vi "Test Bench v15 - TDMS.vi"() -> ()   [LabVIEW 2022 SP3]
uses:
  WhiteNoise.ctl
  <vilib>/Utility/error.llb/DialogType.ctl
  <vilib>/Platform/TimedLoop/XDataNode/timing_clust.ctl
  <vilib>/Platform/TimedLoop/XDataNode/nitl_modes.ctl
  <vilib>/Platform/TimedLoop/XDataNode/wakeup.ctl
  <vilib>/DAQmx/write.llb/DAQmx Write (Analog 2D DBL NChan NSamp).vi
  <vilib>/DAQmx/read.llb/DAQmx Read (Analog 1D DBL 1Chan NSamp).vi
  <vilib>/DAQmx/create/channels.llb/DAQmx Create Channel (AI-Acceleration-Accelerometer).vi
  <vilib>/DAQmx/configure/timing.llb/DAQmx Timing (Sample Clock).vi
  <vilib>/DAQmx/miscellaneous.llb/DAQmx Fill In Error Info.vi
  <vilib>/platform/TimedLoop/XDataNode/XDataNode.xnode
  <vilib>/DAQmx/create/channels.llb/DAQmx Create Channel (AO-Voltage-Basic).vi
  <resource>/objmgr/daqmx.rc
  <vilib>/measure/NI_MABase.lvlib
  <vilib>/Platform/TimedLoop/XDataNode/XDNodeRunTimeDep.lvlib
  <vilib>/Platform/TimedLoop/TimeConversion.llb/rt-milliseconds-to-timestamp.vi
panel:
  in  "stop":bool
  out "x/y":dbl
  out "SampClk.Rate":dbl
  out "Accel. 1 Raw":dbl[](graph)
  in  "Enable Display":bool=TRUE
  in  "Folder to save file to":path=path "C:/Users/LAV-UFSC-2023/Documents/LAV-TCC/Dados-Experimentos/Dados-Bancada-LABVIEW"
  out "Output Signal":dynamicdata(graph)
  in  "Accel. 2":bool
  out "New file path":path
  in  "Signal Output\nControl":enum32{"White Noise", "Harmonic"}(tab)
  in  "White Noise\nParameters":T2={"Seed"=0.0, "Standard Deviation"=0.2, "Reset"=FALSE, "Iterator"=1.0, "Seed"=-1, "Lower Cut-Off"=5.0, "Upper Cut-Off"=350.0} {"Upper Cut-Off" min=5.0 max=350.0 step=10.0; "Lower Cut-Off" min=5.0 max=350.0 step=10.0; "Standard Deviation" min=0.001 max=3.0 step=0.05 format="%0.2p"}
  out "dt White Noise":dbl
  in  "Hamonic\nParameters":T3={"Waveform Type"=0, "Frequency"=10.0, "Amplitude"=0.25} {"Frequency" min=5.0 max=350.0 step=10.0 format="%0.2p"; "Waveform Type" items=["Sine Wave", "Triangle Wave", "Square Wave", "Sawtooth Wave"]; "Amplitude" min=0.001 max=0.3 step=0.05 format="%0.2p"}
  out "dt Harmonic":dbl
  in  "Output":bool=TRUE
  # "Filter"
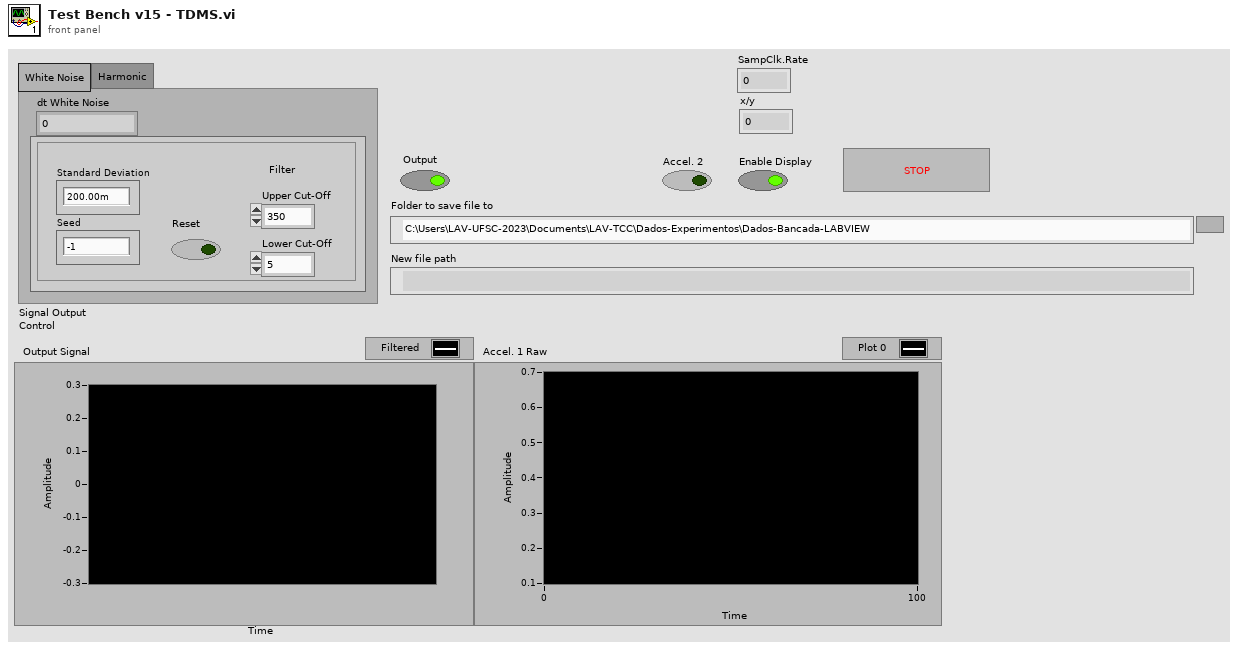
[diagram p1: front panel]
types:
  T1 = typedef "WhiteNoise.ctl" = dbl
  T2 = cluster{"Seed":T1, "Standard Deviation":dbl, "Reset":bool, "Iterator":dbl, "Seed":i8, "Lower Cut-Off":dbl, "Upper Cut-Off":dbl}
  T3 = cluster{"Waveform Type":u16, "Frequency":dbl, "Amplitude":dbl}
  T4 = typedef "DialogType.ctl" = u16
  T5 = enum16{"open", "open or create", "create or replace", "create", "open (read-only)"}
  T6 = typedef "XDNodeRunTimeDep.lvlib/timing_clust.ctl" = cluster{"Expected End [f-1]":u64, "Actual End [f-1]":u64, "Finished Late? [f-1]":bool, "Expected End [i-1]":u64, "Actual End [i-1]":u64, "Finished Late? [i-1]":bool, "Expected Start [i]":u64, "Actual Start [i]":u64, "Expected Start [f]":u64, "Actual Start [f]":u64, "Source Name":string, "Structure Name":string, "Period":i64, "Deadline":i64, "Offset":i64, "Start":i64, "Priority":i32, "Timeout":i32, "Mode":T7, "Wakeup Reason":T8, "Error":errorcluster, "Source Type":string, "Secondary Source Type":string, "Global End Time":u64, "Global Start Time":u64, "Frame Duration":u64, "Iteration Duration":u64, "Assigned CPU":i32, "I/O Scan Engine Mode":u32}
  T7 = typedef "XDNodeRunTimeDep.lvlib/nitl_modes.ctl" = enum32{"No Change", "Process missed periods, maintain original phase", "Discard missed periods, maintain original phase", "Process missed periods, ignore original phase", "Discard missed periods, ignore original phase"}
  T8 = typedef "XDNodeRunTimeDep.lvlib/wakeup.ctl" = enum32{"Normal", "Aborted", "Asynchronous wakeup", "Timing source error", "Timed loop error", "Timeout"}
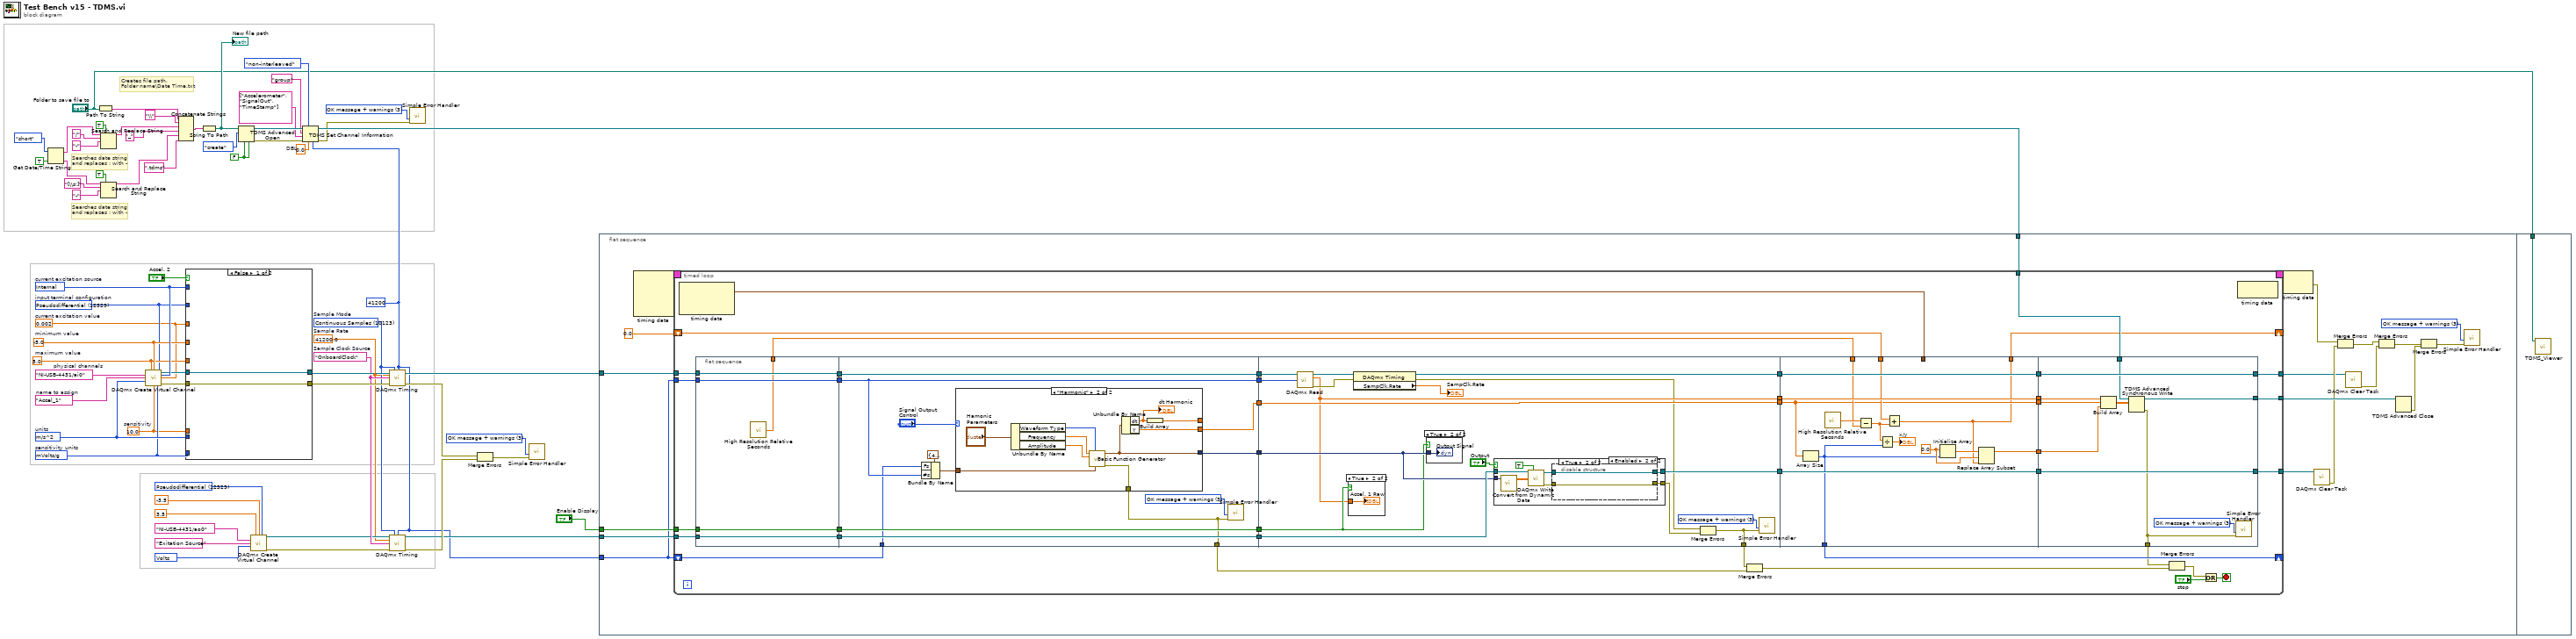
[diagram p0: block diagram]
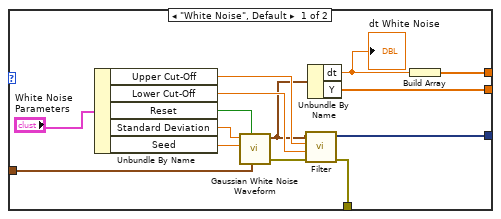
[diagram p2: hidden frame]
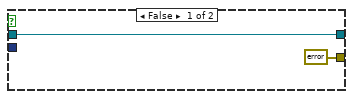
[diagram p5: hidden frame]
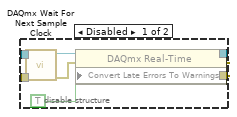
[diagram p6: hidden frame]
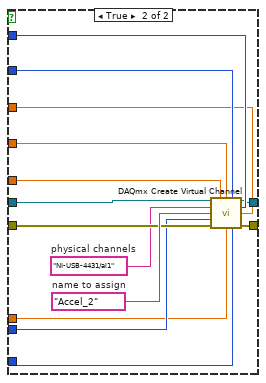
[diagram p7: hidden frame]
diagram:
  w4 = T4 3 items=["no dialog", "OK message", "continue or stop message", "OK message + warnings", "continue/stop + warnings"] ("type of dialog (OK msg:1)")
  w1 = 41200 ("samples per channel")
  w9 = 0.0  # DBL
  w11 = FALSE ("enable asynchronous? (T)")
  w7 = T4 3 items=["no dialog", "OK message", "continue or stop message", "OK message + warnings", "continue/stop + warnings"] ("type of dialog (OK msg:1)")
  w51 = 12529 items=["Default"=-1, "RSE"=10083, "Differential"=10106, "Pseudodifferential"=12529] ("output terminal configuration")
  w49 = 10348 items=["Volts"=10348, "From Custom Scale"=10065] ("units")
  w55 = 12509 items=["mVolts/g"=12509, "Volts/g"=12510]  # sensitivity units
  w46 = 10.0  # sensitivity
  w54 = 0.002  # current excitation value
  w62 = 10200 items=["Internal"=10200, "External"=10167, "None"=10230]  # current excitation source
  w56 = tag "NI-USB-4431/ai0"  # physical channels
  w43 = tag "OnboardClock"  # Sample Clock Source
  w6 = 41200.0  # Sample Rate
  w42 = 10123 items=["Finite Samples"=10178, "Continuous Samples"=10123, "Hardware Timed Single Point"=12522]  # Sample Mode
  w58 = 12529 items=["default"=-1, "RSE"=10083, "NRSE"=10078, "Differential"=10106, "Pseudodifferential"=12529]  # input terminal configuration
  w61 = -5.0  # minimum value
  w60 = 5.0  # maximum value
  w64 = "Accel_1"  # name to assign
  w59 = 12470 items=["g"=10186, "m/s^2"=12470, "in/s^2"=12471, "From Custom Scale"=10065]  # units
  # "Searches date string\nand replaces : with -"
  # "Searches date string\nand replaces : with -"
  # "Creates file path.\nFolder name\\Date Time.txt"
  n1 = Get Date/Time String(date format (0)=enum16{"short", "long", "abbreviated"}."short", want seconds? (F)=TRUE) -> (date string=w19:string, time string=w32:string)  [unwired: 1 in]
  n2 = Path To String(path="Folder to save file to") -> (string=w27:string)
  n3 = Search and Replace String(replace all?=TRUE ("replace all? (F)"), input string=w19, search string="/" ("replace string (\"\")"), replace string="-" ("replace string (\"\")")) -> (result string=w18:string)  [unwired: 4 in, 3 out]
  n4 = Search and Replace String(replace all?=TRUE ("replace all? (F)"), input string=w32, search string="[\\s:]" ("replace string (\"\")"), replace string="-" ("replace string (\"\")")) -> (result string=w25:string)  [unwired: 4 in, 3 out]
  n5 = call-poly <vilib>:"DAQmx Create Virtual Channel.vi"("maximum value"=w60, "minimum value"=w61, "input terminal configuration"=w58, "physical channels"=w56, "current excitation source"=w62, "name to assign"=w64, "current excitation value"=w54, "units"=w59, "sensitivity"=w46, "sensitivity units"=w55) -> ("task out"=w57:refnum<k21>, "error out"=w63:errorcluster)  [unwired: 4 in]
  n6 = Concatenate Strings(w27, "\\" ("string"), w18, "_" ("string"), w25, ".tdms" ("string")) -> (w23:string)
  n7 = case shown="False" "Accel. 2" {
    tunnel: w63 -> [w66 w79]
    tunnel: w62 -> [_ w78]
    tunnel: w61 -> [_ w77]
    tunnel: w60 -> [_ w76]
    tunnel: w59 -> [_ w75]
    tunnel: w58 -> [_ w74]
    tunnel: w57 -> [w65 w73]
    tunnel: w55 -> [_ w71]
    tunnel: w54 -> [_ w70]
    tunnel: w46 -> [_ w69]
    tunnel: [w66 w68] -> w45
    tunnel: [w65 w67] -> w44
    frame False {
    }
    frame True {
      w72 = tag "NI-USB-4431/ai1"  # physical channels
      w80 = "Accel_2"  # name to assign
      n8 = call-poly <vilib>:"DAQmx Create Virtual Channel.vi"("task in"=w73, "maximum value"=w76, "minimum value"=w77, "input terminal configuration"=w74, "physical channels"=w72, "current excitation source"=w78, "name to assign"=w80, "current excitation value"=w70, "units"=w75, "error in"=w79, "sensitivity"=w69, "sensitivity units"=w71) -> ("task out"=w67:refnum<k21>, "error out"=w68:errorcluster)  [unwired: 2 in]
    }
  }
  n9 = String To Path(string=w23) -> (path=w36:path)
  "New file path" <- w36
  n10 = TDMS Advanced Open(4:w11, 6:w11, 10:T5."create" ("operation (0:open)"), 11:w36) -> (0:w15:errorcluster, 3:w14:refnum<k34>)  [unwired: 1 in, 1 out]
  n11 = call-poly <vilib>:"DAQmx Create Virtual Channel.vi"("maximum value"=3.5, "minimum value"=-3.5, "output terminal configuration"=w51, "physical channels"=tag "NI-USB-4431/ao0", "name to assign"="Exitation Source", "units"=w49) -> ("task out"=w40:refnum<k21>, "error out"=w41:errorcluster)  [unwired: 8 in]
  n12 = TDMS Set Channel Information(4:w1, 6:w9, 7:enum16{"non-interleaved", "interleaved"}."non-interleaved" ("data layout (0:non-interleaved)"), 8:w15, 9:string[] ["Accelerometer", "SignalOut", "TimeStamp"] ("channel name(s)"), 10:"group" ("group name (Untitled)"), 11:w14) -> (0:w8:errorcluster, 3:w35:refnum<k34>)
  n13 = call-poly <vilib>:"DAQmx Timing.vi"("task/channels in"=w44, "sample mode"=w42, "samples per channel"=w1, "rate"=w6, "source"=w43, "error in"=w45) -> ("task out"=w3:refnum<k21>, "error out"=w48:errorcluster)  [unwired: 8 in]
  n14 = call-poly <vilib>:"DAQmx Timing.vi"("task/channels in"=w40, "sample mode"=w42, "samples per channel"=w1, "rate"=w6, "source"=w43, "error in"=w41) -> ("task out"=w38:refnum<k21>, "error out"=w39:errorcluster)  [unwired: 8 in]
  n15 = call <vilib>:"Simple Error Handler.vi"("type of dialog (OK msg:1)"=w7, "error in (no error)"=w8) -> ()  [unwired: 3 in, 5 out]
  n16 = Merge Errors(w48, w39) -> (w2:errorcluster)
  n17 = call <vilib>:"Simple Error Handler.vi"("type of dialog (OK msg:1)"=w4, "error in (no error)"=w2) -> ()  [unwired: 3 in, 5 out]
  n18 = flat-sequence {
    tunnel: w38 -> [w96]
    tunnel: w3 -> [w94]
    tunnel: w35 -> [w93]
    tunnel: "Enable Display" -> [w91]
    tunnel: w1 -> [w81]
    tunnel: "Folder to save file to" -> [w250]
    frame #0 {
      w97 = T4 3 items=["no dialog", "OK message", "continue or stop message", "OK message + warnings", "continue/stop + warnings"] ("type of dialog (OK msg:1)")
      n19 = node-c288() -> (w99:T6)  [unwired: 4 in]
      n20 = timed-loop {
        tunnel: w96 -> [w139]
        tunnel: [w137] -> w95
        tunnel: w94 -> [w138]
        tunnel: [w136] -> w88
        tunnel: w93 -> [w112]
        tunnel: [w133] -> w92
        tunnel: w91 -> [w135]
        shift-right: [w108] -> _
        shift-left: w81 -> [w117]
        tunnel: w81 -> [w120]
        timing: w99 -> [_]
        timing-out: [_] -> w98
        shift-right: [w107] -> _
        shift-left: 0.0 -> [w110]
        stop <- w118 stop-if-true
        n21 = node-c288() -> (w111:timestamp)  [unwired: 1 in, 2 out]
        n22 = flat-sequence {
          tunnel: w135 -> [w146]
          tunnel: w138 -> [w147]
          tunnel: w139 -> [w148]
          tunnel: [w148] -> w134
          tunnel: [w147] -> w132
          tunnel: [w146] -> w123
          tunnel: w120 -> [w145]
          tunnel: [w145] -> w119
          tunnel: [w144] -> w109
          tunnel: w134 -> [w156]
          tunnel: [w157] -> w131
          tunnel: [w153] -> w129
          tunnel: w132 -> [w157]
          tunnel: [w156] -> w127
          tunnel: [w154] -> w125
          tunnel: [w155] -> w124
          tunnel: w123 -> [w154]
          tunnel: [w152] -> w121
          tunnel: w119 -> [w152]
          tunnel: w117 -> [w151]
          tunnel: [w150] -> w103
          tunnel: w131 -> [w193]
          tunnel: [w189] -> w130
          tunnel: w129 -> [w201]
          tunnel: [w201] -> w128
          tunnel: w127 -> [w199]
          tunnel: [w198] -> w126
          tunnel: w125 -> [w194]
          tunnel: w124 -> [w197]
          tunnel: [w192] -> w122
          tunnel: w121 -> [w191]
          tunnel: [w185] -> w104
          tunnel: w130 -> [w234]
          tunnel: w128 -> [w230]
          tunnel: w126 -> [w236]
          tunnel: w122 -> [w235]
          tunnel: [w236] -> w116
          tunnel: [w235] -> w115
          tunnel: [w234] -> w114
          tunnel: [w230] -> w113
          tunnel: w111 -> [_]
          tunnel: w110 -> [w231]
          tunnel: w109 -> [w232]
          tunnel: [w223] -> w108
          tunnel: [w225] -> w107
          tunnel: [w226] -> w106
          tunnel: [w242] -> w133
          tunnel: [w245] -> w136
          tunnel: [w246] -> w137
          tunnel: w116 -> [w246]
          tunnel: w115 -> [w245]
          tunnel: w114 -> [w240]
          tunnel: w113 -> [w241]
          tunnel: w112 -> [w243]
          tunnel: w106 -> [w239]
          tunnel: [w237] -> w100
          frame #0 {
            n23 = call <vilib>:"High Resolution Relative Seconds.vi"() -> ("relative seconds"=w144:dbl)
          }
          frame #1 {
            w149 = T4 3 items=["no dialog", "OK message", "continue or stop message", "OK message + warnings", "continue/stop + warnings"] ("type of dialog (OK msg:1)")
            n24 = Bundle By Name(cluster=cluster{"Fs":dbl, "#s":dbl} {"Fs"=41200.0, "#s"=41200.0} ("sampling info"), "Fs"=w151, "#s"=w152) -> (w159:cluster{"Fs":dbl, "#s":dbl})
            n25 = case shown="\"Harmonic\"" "Signal Output\nControl" {
              tunnel: w159 -> [w172 w183]
              tunnel: [w164 w178] -> _
              tunnel: [w163 w177] -> w155
              tunnel: [w162 w176] -> w153
              tunnel: [w161 w175] -> w150
              frame "White Noise", Default {
                n26 = Unbundle By Name("White Noise\nParameters") -> ("Upper Cut-Off"=w168:dbl, "Lower Cut-Off"=w167:dbl, "Reset"=w169:bool, "Standard Deviation"=w170:dbl, "Seed"=w171:T1)
                n27 = call <vilib>:"Gaussian White Noise Waveform.vi"("sampling info"=w172, "reset signal"=w169, "seed"=w171, "standard deviation"=w170) -> ("error out"=w174:errorcluster, "signal out"=w166:waveform(dbl))  [unwired: 6 in]
                n28 = call "Filter"("error in (no error)"=w174, "Lower Cut-Off"=w167, "Upper Cut-Off"=w168, "Signal"=w166) -> ("error out"=w161:errorcluster, "Filtered Signal"=w163:dynamicdata)  [unwired: 6 in]
                n29 = Unbundle By Name(w166) -> ("dt"=w165:dbl, "Y"=w162:dbl[])
                "dt White Noise" <- w165
                n30 = Build Array(w165) -> (w164:dbl[])
              }
              frame "Harmonic" {
                n31 = Unbundle By Name("Hamonic\nParameters") -> ("Waveform Type"=w182:u16, "Frequency"=w181:dbl, "Amplitude"=w180:dbl)
                n32 = call <vilib>:"Basic Function Generator.vi"("sampling info"=w183, "signal type"=w182, "amplitude"=w180, "frequency"=w181) -> ("error out"=w175:errorcluster, "signal out"=w177:waveform(dbl))  [unwired: 5 in, 1 out]
                n33 = Unbundle By Name(w177) -> ("dt"=w179:dbl, "Y"=w176:dbl[])
                "dt Harmonic" <- w179
                n34 = Build Array(w179) -> (w178:dbl[])
              }
            }
            n35 = call <vilib>:"Simple Error Handler.vi"("type of dialog (OK msg:1)"=w149, "error in (no error)"=w150) -> ()  [unwired: 3 in, 5 out]
          }
          frame #2 {
            w188 = T4 3 items=["no dialog", "OK message", "continue or stop message", "OK message + warnings", "continue/stop + warnings"] ("type of dialog (OK msg:1)")
            n36 = call-poly <vilib>:"DAQmx Read.vi"("task/channels in"=w193, "number of samples per channel"=w191) -> ("task out"=w195:refnum<k21>, "data"=w189:dbl[], "error out"=w196:errorcluster)  [unwired: 11 in]
            n37 = case shown="True" w194 {
              tunnel: w189 -> [_ w202]
              frame False {
              }
              frame True {
                "Accel. 1 Raw" <- w202
              }
            }
            n38 = property class="DAQmx Timing"(reference=w195, error in=w196) -> (reference out=w192:refnum<k21>, error out=w187:errorcluster, "SampClk.Rate"=→"SampClk.Rate":dbl)
            n39 = case shown="True" w194 {
              tunnel: w197 -> [_ w203]
              frame False {
              }
              frame True {
                "Output Signal" <- w203
              }
            }
            n40 = case shown="True" "Output" {
              tunnel: w199 -> [w205 w213]
              tunnel: [errorcluster {"status"=FALSE, "code"=0, "source"=""} ("error out") w209] -> w186
              tunnel: [w205 w210] -> w198
              tunnel: w197 -> [_ w208]
              frame False {
              }
              frame True {
                n41 = call "Convert from Dynamic Data"("Dynamic Data Type"=w208) -> ("Array"=w207:dbl[][])  [unwired: 3 in]
                n42 = call-poly <vilib>:"DAQmx Write.vi"("task/channels in"=w213, "auto start"=TRUE, "data"=w207) -> ("task out"=w212:refnum<k21>, "error out"=w211:errorcluster)  [unwired: 10 in, 1 out]
                n43 = disable-structure shown="Enabled" {
                  disable-tunnel: w212 -> [w220 w221]
                  disable-tunnel: w211 -> [w219 w222]
                  disable-tunnel: [w217 w221] -> w210
                  disable-tunnel: [w216 w222] -> w209
                  frame Disabled {
                    n44 = call <vilib>:"DAQmx Wait For Next Sample Clock.vi"("task/channels in"=w220, "error in"=w219) -> ("task out"=w218:refnum<k21>, "error out"=w215:errorcluster)  [unwired: 11 in, 1 out]
                    n45 = property class="DAQmx Real-Time"(reference=w218, error in=w215, "Convert Late Errors To Warnings"=TRUE ("ConvLateErrorsToWarnings")) -> (reference out=w217:refnum<k21>, error out=w216:errorcluster)
                  }
                  frame Enabled {
                  }
                }
              }
            }
            n46 = Merge Errors(w187, w186) -> (w185:errorcluster)
            n47 = call <vilib>:"Simple Error Handler.vi"("type of dialog (OK msg:1)"=w188, "error in (no error)"=w185) -> ()  [unwired: 3 in, 5 out]
          }
          frame #3 {
            w227 = 0.0 ("element")
            n48 = Array Size(array=w230) -> (size(s)=w223:i32)
            n49 = call <vilib>:"High Resolution Relative Seconds.vi"() -> ("relative seconds"=w233:dbl)
            n50 = Subtract(x=w233, y=w232) -> (x-y=w229:dbl)
            n51 = Divide(x=w229, y=w223) -> (x/y=→"x/y":dbl)
            n52 = Add(x=w231, y=w229) -> (x+y=w225:dbl)
            n53 = Initialize Array(w227, w223) -> (w228:dbl[])
            n54 = Replace Array Subset(array=w228, new element=w225, index=w227) -> (w226:dbl[])
          }
          frame #4 {
            w238 = T4 3 items=["no dialog", "OK message", "continue or stop message", "OK message + warnings", "continue/stop + warnings"] ("type of dialog (OK msg:1)")
            n55 = Build Array(w240, w241, w239) -> (w244:dbl[][])
            n56 = TDMS Advanced Synchronous Write(10:w244, 11:w243) -> (0:w237:errorcluster, 3:w242:refnum<k34>)  [unwired: 1 in]
            n57 = call <vilib>:"Simple Error Handler.vi"("type of dialog (OK msg:1)"=w238, "error in (no error)"=w237) -> ()  [unwired: 3 in, 5 out]
          }
        }
        n58 = Merge Errors(w104, w103) -> (w102:errorcluster)
        n59 = Merge Errors(w100, w102) -> (w101:errorcluster)
        n60 = Or(x=w101, y="stop") -> (x .or. y?=w118:bool)
        n61 = node-c288() -> ()  [unwired: 1 in, 1 out]
      }
      n62 = node-c288(w98) -> (w83:errorcluster)
      n63 = call <vilib>:"DAQmx Clear Task.vi"("task in"=w95) -> ("error out"=w90:errorcluster)  [unwired: 14 in]
      n64 = Merge Errors(w83, w90) -> (w87:errorcluster)
      n65 = call <vilib>:"DAQmx Clear Task.vi"("task in"=w88) -> ("error out"=w86:errorcluster)  [unwired: 14 in]
      n66 = Merge Errors(w87, w86) -> (w85:errorcluster)
      n67 = TDMS Advanced Close(11:w92) -> (0:w89:errorcluster)  [unwired: 3 in, 1 out]
      n68 = Merge Errors(w85, w89) -> (w84:errorcluster)
      n69 = call <vilib>:"Simple Error Handler.vi"("type of dialog (OK msg:1)"=w97, "error in (no error)"=w84) -> ()  [unwired: 3 in, 5 out]
    }
    frame #1 {
      n70 = call "TDMS_Viewer.vi"("Data Directory"=w250) -> ()  [unwired: 11 in]
    }
  }
